vi "InsertNewPBMeasurement.vi"(10 "Message":T1, 11 "Table in":refnum<vi>) -> ()   [LabVIEW 2013, in "main.lvlib"]
uses:
  main.lvlib
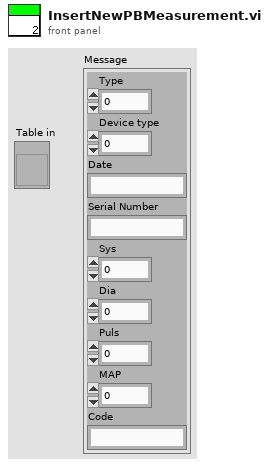
[diagram p1: front panel]
types:
  T1 = cluster{"Type":i32, "Device type":i32, "Date":string, "Serial Number":string, "Sys":i32, "Dia":i32, "Puls":i32, "MAP":i32, "Code":string}
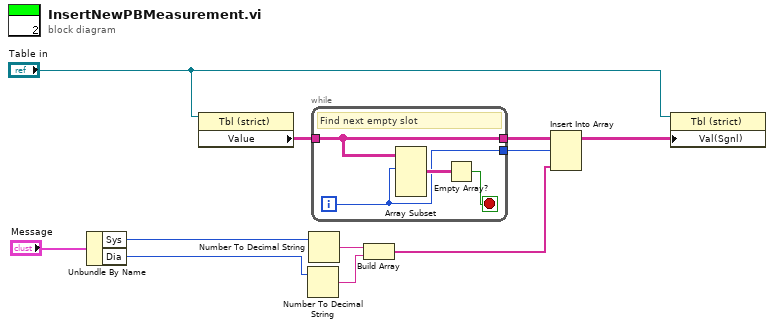
[diagram p0: block diagram]
diagram:
  n1 = Unbundle By Name("Message") -> ("Sys"=w2:i32, "Dia"=w1:i32)
  n2 = property class="Tbl (strict)"(reference="Table in") -> ("Value"=w4:string[][])  [unwired: 1 in, 2 out]
  n3 = Number To Decimal String(number=w1) -> (decimal integer string=w7:string)  [unwired: 1 in]
  n4 = Number To Decimal String(number=w2) -> (decimal integer string=w6:string)  [unwired: 1 in]
  n5 = while {
    tunnel: w4 -> [w14]
    tunnel: [w14] -> w8
    tunnel: [w12] -> w11
    i -> [w12]
    stop <- w13 stop-if-true
    # "Find next empty slot"
    n6 = Array Subset(array=w14, index (row)=w12) -> (w15:string[][])  [unwired: 3 in]
    n7 = Empty Array?(array=w15) -> (empty?=w13:bool)
  }
  n8 = Build Array(w6, w7) -> (w10:string[])
  n9 = Insert Into Array(array=w8, index (row)=w11, new element=w10) -> (w9:string[][])  [unwired: 1 in]
  n10 = property class="Tbl (strict)"(reference="Table in", "Val(Sgnl)"=w9) -> ()  [unwired: 1 in, 2 out]
